vi "ScaleWayPoints_USB7855R.vi"(8 "AO Calibration Constants":cluster{"LSB Weight":u32, "Offset":i32}[](array[cluster]), 11 "WayPointCluster":T2) -> (0 "FPGA Way Points":i16[](array[numeric]), 2 "VelScallerCluster":T1, 3 ".not. x?":bool)   [LabVIEW 2023]
uses:
  TypeDefs/WayPointCluster.ctl
  TypeDefs/VelScallerCluster.ctl
  User_Vi/Settings.vi
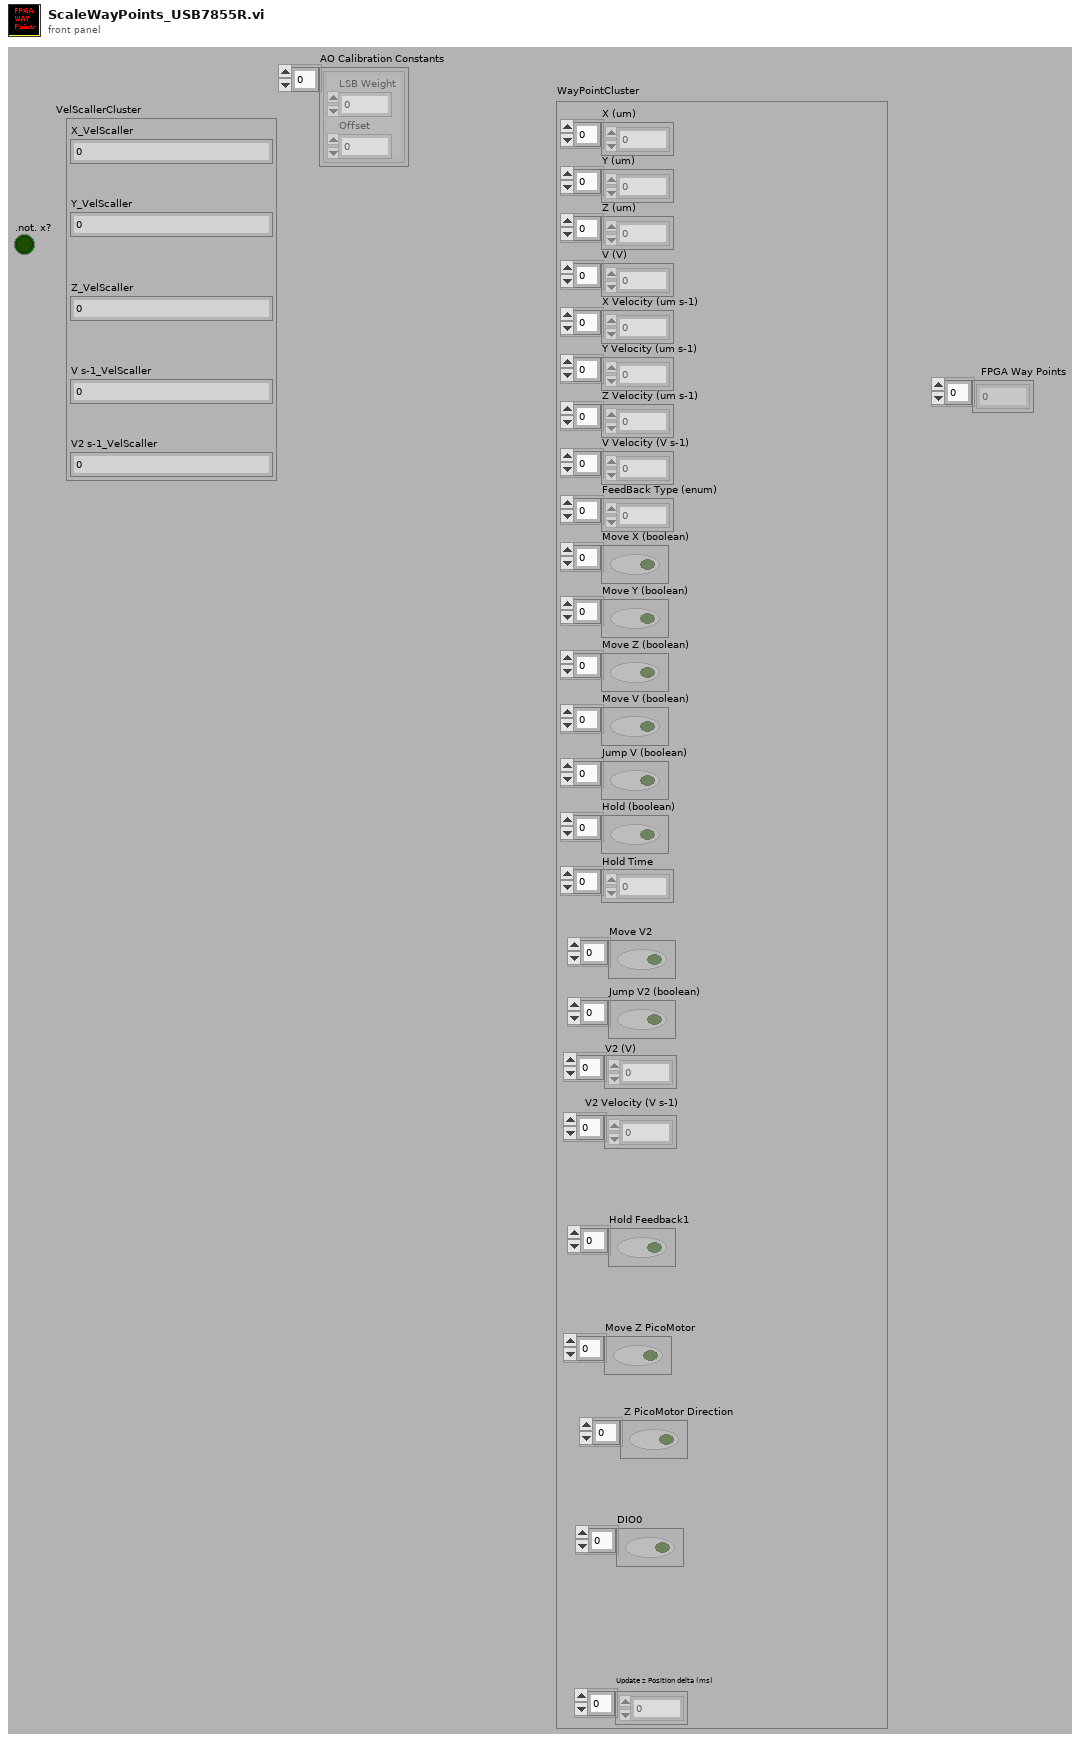
[diagram p1: front panel]
types:
  T1 = typedef "VelScallerCluster.ctl" = cluster{"X_VelScaller":i32, "Y_VelScaller":i32, "Z_VelScaller":i32, "V s-1_VelScaller":i32, "V2 s-1_VelScaller":i32}
  T2 = typedef "WayPointCluster.ctl" = cluster{"X (um)":dbl[], "Y (um)":dbl[], "Z (um)":dbl[], "V (V)":dbl[], "X Velocity (um s-1)":dbl[], "Y Velocity (um s-1)":dbl[], "Z Velocity (um s-1)":dbl[], "V Velocity (V s-1)":dbl[], "FeedBack Type (enum)":u16[], "Move X (boolean)":bool[], "Move Y (boolean)":bool[], "Move Z (boolean)":bool[], "Move V (boolean)":bool[], "Jump V (boolean)":bool[], "Hold (boolean)":bool[], "Hold Time":u32[], "V2 (V)":dbl[], "Move V2":bool[], "V2 Velocity (V s-1)":dbl[], "Jump V2 (boolean)":bool[], "Update z Position delta (ms)":i16[], "Hold Feedback1":bool[], "Move Z PicoMotor":bool[], " Z PicoMotor Direction":bool[], "DIO0":bool[]}
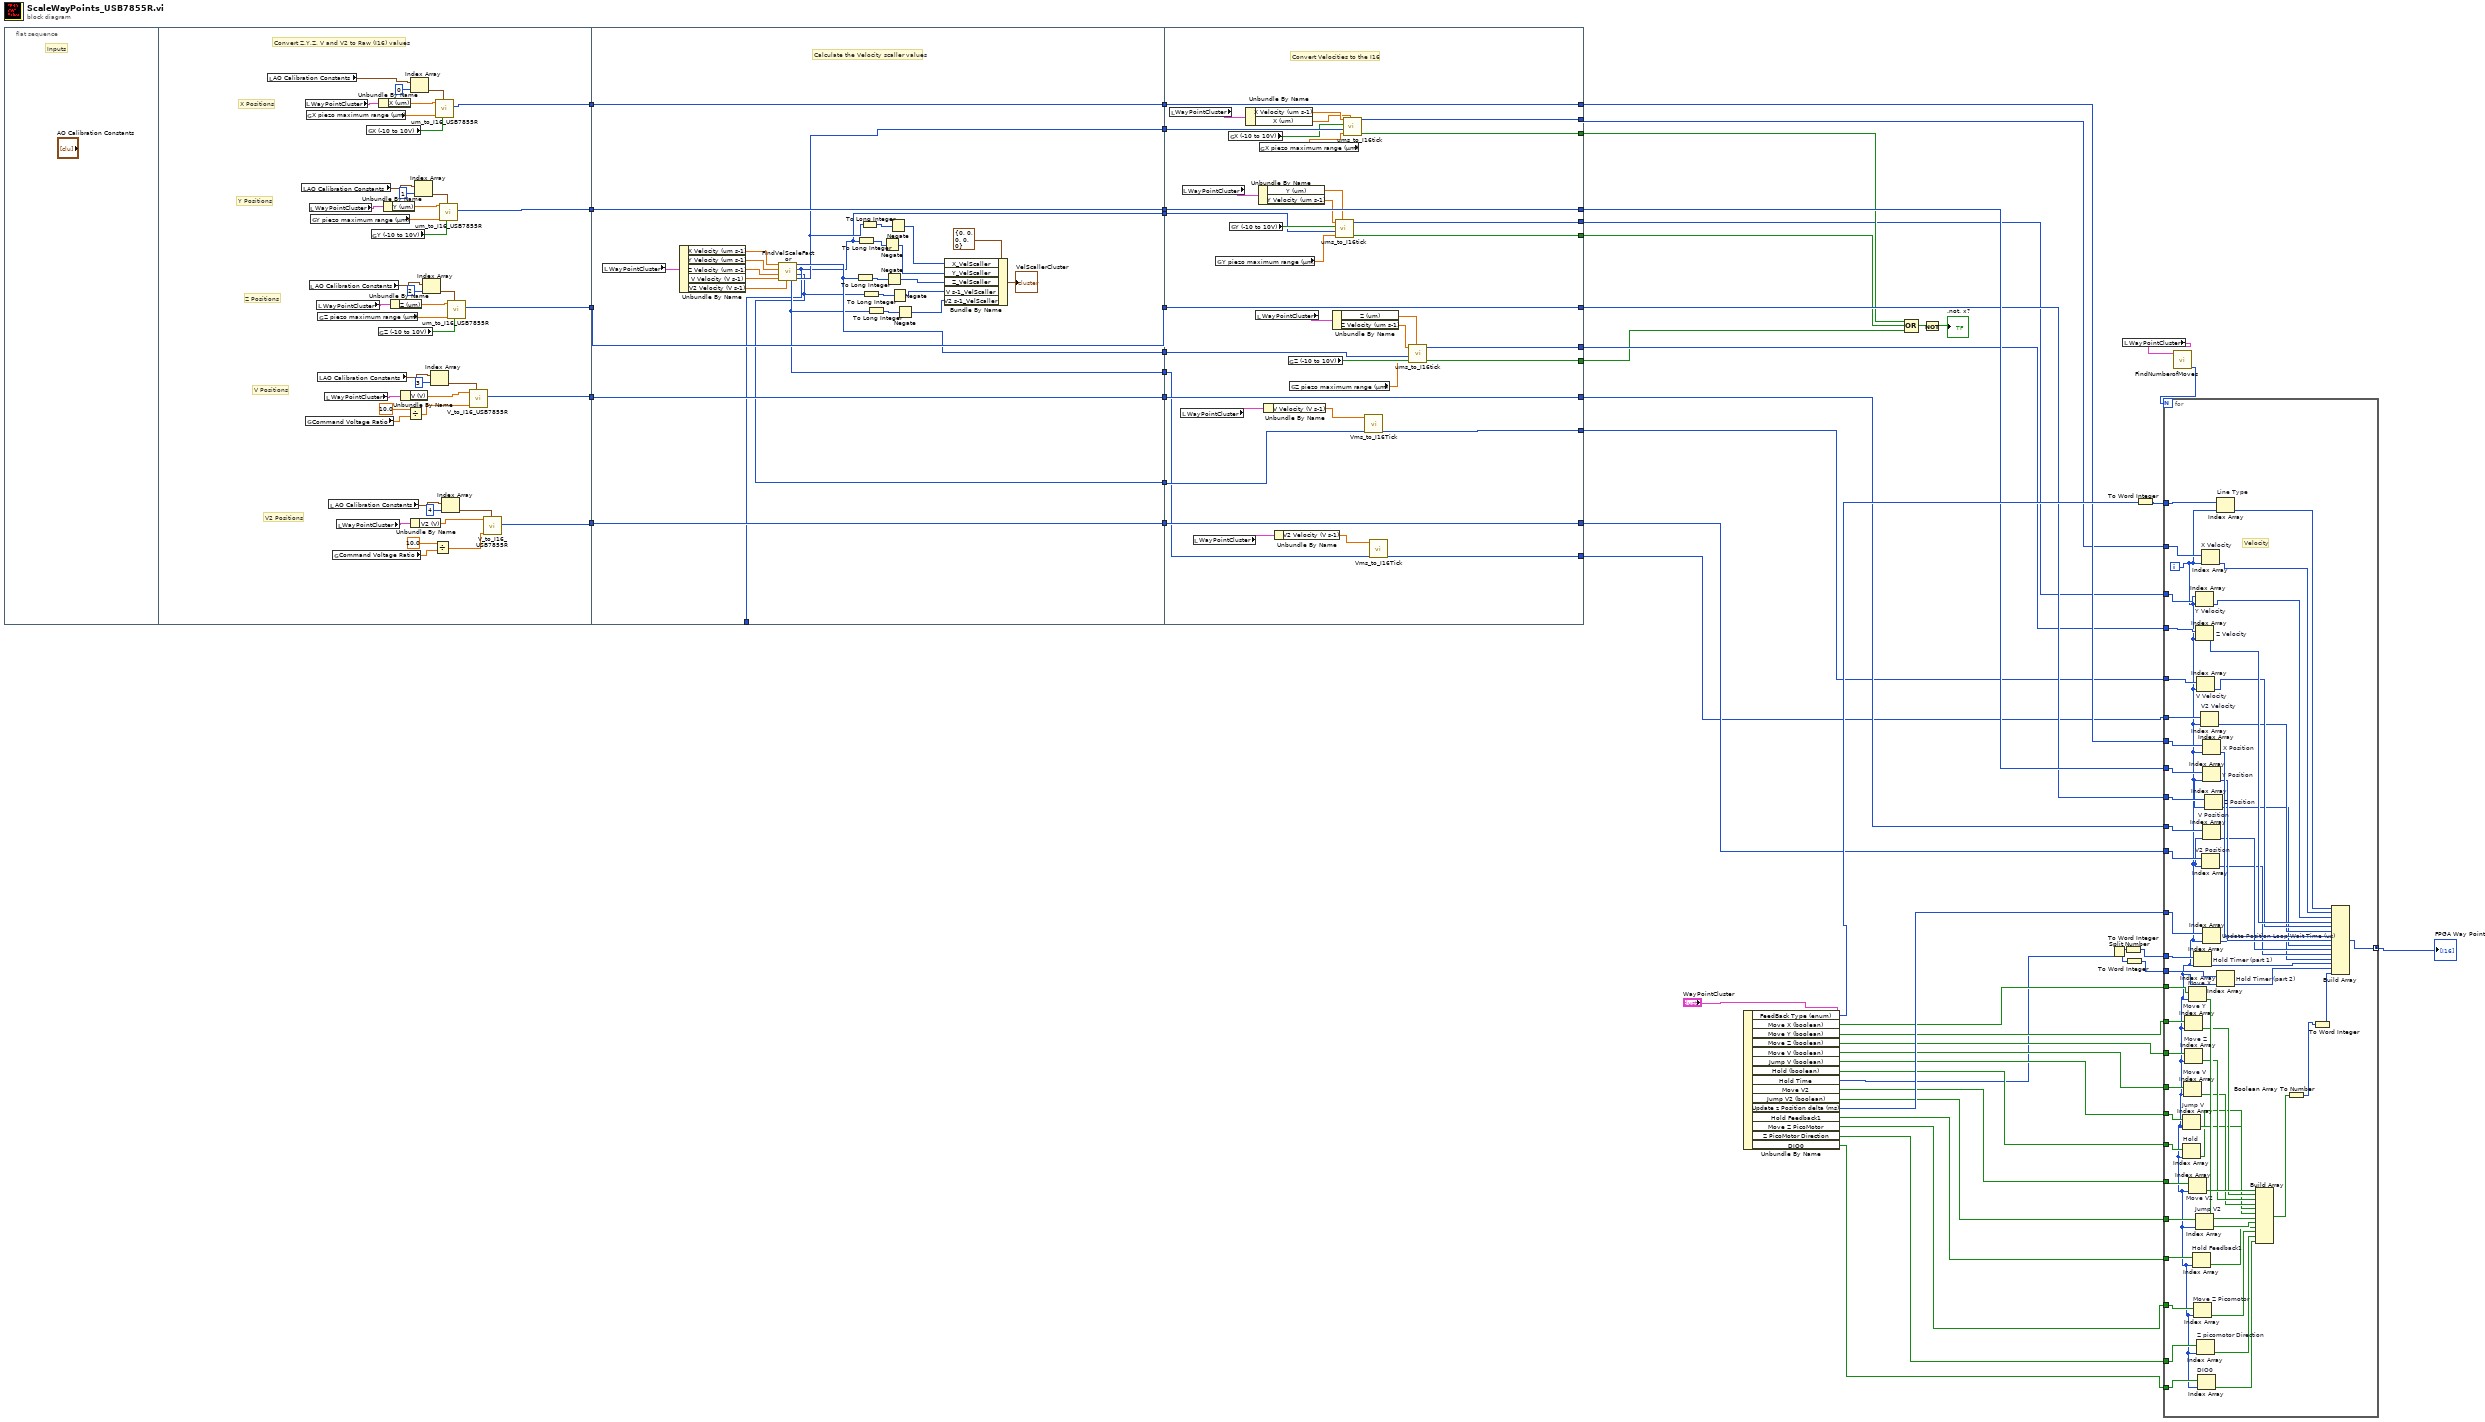
[diagram p0: block diagram]
diagram:
  n1 = flat-sequence {
    tunnel: [w96] -> w25
    tunnel: [w81] -> w24
    tunnel: [w73] -> w23
    tunnel: [w61] -> w22
    tunnel: [w55] -> w21
    tunnel: w25 -> [w124]
    tunnel: w24 -> [w123]
    tunnel: w23 -> [w122]
    tunnel: w22 -> [w121]
    tunnel: w21 -> [w120]
    tunnel: [w98] -> _
    tunnel: [w124] -> w20
    tunnel: [w123] -> w19
    tunnel: [w122] -> w18
    tunnel: [w121] -> w17
    tunnel: [w120] -> w16
    tunnel: [w119] -> w15
    tunnel: [w118] -> w14
    tunnel: [w99] -> w11
    tunnel: [w98] -> w10
    tunnel: [w97] -> w4
    tunnel: [w157] -> w26
    tunnel: [w158] -> w27
    tunnel: [w159] -> w28
    tunnel: [w160] -> w29
    tunnel: [w161] -> w30
    tunnel: w20 -> [w161]
    tunnel: w19 -> [w160]
    tunnel: w18 -> [w159]
    tunnel: w17 -> [w158]
    tunnel: w16 -> [w157]
    tunnel: w15 -> [w135]
    tunnel: w14 -> [w128]
    tunnel: [w156] -> w13
    tunnel: [w155] -> w12
    tunnel: w11 -> [w154]
    tunnel: w10 -> [w143]
    tunnel: [w142] -> w8
    tunnel: [w141] -> w9
    tunnel: [w134] -> w6
    tunnel: [w133] -> w7
    tunnel: [w132] -> w5
    tunnel: w4 -> [w129]
    tunnel: [w127] -> w3
    frame #0 {
      # "Inputs"
    }
    frame #1 {
      # "V2 Positions"
      # "V Positions"
      # "Z Positions"
      # "Y Positions"
      # "X Positions"
      # "Convert Z,Y,Z, V and V2 to Raw (I16) values"
      n2 = local read "AO Calibration Constants"() -> (w92:cluster{"LSB Weight":u32, "Offset":i32}[])
      n3 = local read "AO Calibration Constants"() -> (w85:cluster{"LSB Weight":u32, "Offset":i32}[])
      n4 = local read "WayPointCluster"() -> (w94:T2)
      n5 = global read "Settings.vi" "Command Voltage Ratio"() -> (w63:dbl)
      n6 = global read "Settings.vi" "X piezo maximum range (µm)"() -> (w95:dbl)
      n7 = local read "WayPointCluster"() -> (w83:T2)
      n8 = local read "AO Calibration Constants"() -> (w77:cluster{"LSB Weight":u32, "Offset":i32}[])
      n9 = global read "Settings.vi" "Y piezo maximum range (µm)"() -> (w82:dbl)
      n10 = local read "WayPointCluster"() -> (w79:T2)
      n11 = local read "AO Calibration Constants"() -> (w71:cluster{"LSB Weight":u32, "Offset":i32}[])
      n12 = global read "Settings.vi" "Z piezo maximum range (µm)"() -> (w80:dbl)
      n13 = local read "WayPointCluster"() -> (w70:T2)
      n14 = local read "AO Calibration Constants"() -> (w68:cluster{"LSB Weight":u32, "Offset":i32}[])
      n15 = global read "Settings.vi" "Command Voltage Ratio"() -> (w58:dbl)
      n16 = local read "WayPointCluster"() -> (w69:T2)
      n17 = global read "Settings.vi" "X (-10 to 10V)"() -> (w89:bool)
      n18 = global read "Settings.vi" "Y (-10 to 10V)"() -> (w88:bool)
      n19 = global read "Settings.vi" "Z (-10 to 10V)"() -> (w74:bool)
      n20 = Unbundle By Name(w94) -> ("X (um)"=w93:dbl[])
      n21 = Unbundle By Name(w83) -> ("Y (um)"=w84:dbl[])
      n22 = Unbundle By Name(w79) -> ("Z (um)"=w78:dbl[])
      n23 = Unbundle By Name(w70) -> ("V (V)"=w65:dbl[])
      n24 = Divide(x=10.0 ("Max/Min Value [V]"), y=w63) -> (x/y=w62:dbl)
      n25 = Index Array(array=w92, index=0) -> (element=w90:cluster{"LSB Weight":u32, "Offset":i32})
      n26 = Unbundle By Name(w69) -> ("V2 (V)"=w59:dbl[])
      n27 = Index Array(array=w85, index=1) -> (element=w87:cluster{"LSB Weight":u32, "Offset":i32})
      n28 = Index Array(array=w77, index=2) -> (element=w75:cluster{"LSB Weight":u32, "Offset":i32})
      n29 = Index Array(array=w71, index=3) -> (element=w66:cluster{"LSB Weight":u32, "Offset":i32})
      n30 = Divide(x=10.0 ("Max/Min Value [V]"), y=w58) -> (x/y=w56:dbl)
      n31 = call "um_to_I16_USB7855R.vi"("-10 to 10V?"=w89, "Calibration Constant"=w90, "Max Value [um]"=w95, "Input"=w93) -> ("Array"=w96:i16[])  [unwired: 7 in]
      n32 = call "um_to_I16_USB7855R.vi"("-10 to 10V?"=w88, "Calibration Constant"=w87, "Max Value [um]"=w82, "Input"=w84) -> ("Array"=w81:i16[])  [unwired: 7 in]
      n33 = Index Array(array=w68, index=4) -> (element=w60:cluster{"LSB Weight":u32, "Offset":i32})
      n34 = call "um_to_I16_USB7855R.vi"("-10 to 10V?"=w74, "Calibration Constant"=w75, "Max Value [um]"=w80, "Input"=w78) -> ("Array"=w73:i16[])  [unwired: 7 in]
      n35 = call "V_to_I16_USB7855R.vi"("Calibration Constant"=w66, "Max/Min Value [V]"=w62, "Input"=w65) -> ("16bit integer"=w61:i16[])  [unwired: 8 in]
      n36 = call "V_to_I16_USB7855R.vi"("Calibration Constant"=w60, "Max/Min Value [V]"=w56, "Input"=w59) -> ("16bit integer"=w55:i16[])  [unwired: 8 in]
    }
    frame #2 {
      # "Calculate the Velocity scaller values"
      n37 = local read "WayPointCluster"() -> (w117:T2)
      n38 = Unbundle By Name(w117) -> ("X Velocity (um s-1)"=w116:dbl[], "Y Velocity (um s-1)"=w115:dbl[], "Z Velocity (um s-1)"=w114:dbl[], "V Velocity (V s-1)"=w113:dbl[], "V2 Velocity (V s-1)"=w112:dbl[])
      n39 = call "FindVelScaleFactor.vi"("V2 Velocity [V s-1]"=w112, "V Velocity [V s-1]"=w113, "Z Velocity [um s-1]"=w114, "Y Velocity [um s-1]"=w115, "X Velocity [um s-1]"=w116) -> ("X_VelScaller"=w99:u32, "V s-1_VelScaller"=w97:u32, "Y_VelScaller"=w98:u32, "Z_VelScaller"=w119:u32, "V2 s-1_VelScaller"=w118:u32)  [unwired: 2 in]
      n40 = To Long Integer(number=w119) -> (32bit integer=w104:i32)
      n41 = To Long Integer(number=w98) -> (32bit integer=w103:i32)
      n42 = To Long Integer(number=w99) -> (32bit integer=w101:i32)
      n43 = To Long Integer(number=w97) -> (32bit integer=w102:i32)
      n44 = To Long Integer(number=w118) -> (32bit integer=w105:i32)
      n45 = Negate(x=w103) -> (-x=w108:i32)
      n46 = Negate(x=w104) -> (-x=w109:i32)
      n47 = Negate(x=w101) -> (-x=w106:i32)
      n48 = Negate(x=w102) -> (-x=w107:i32)
      n49 = Negate(x=w105) -> (-x=w110:i32)
      n50 = Bundle By Name(cluster=T1 {"X_VelScaller"=0, "Y_VelScaller"=0, "Z_VelScaller"=0, "V s-1_VelScaller"=0, "V2 s-1_VelScaller"=0} ("VelScallerCluster"), "X_VelScaller"=w106, "Y_VelScaller"=w108, "Z_VelScaller"=w109, "V s-1_VelScaller"=w107, "V2 s-1_VelScaller"=w110) -> (→"VelScallerCluster":T1)
    }
    frame #3 {
      # "Convert Velocities to the I16"
      n51 = local read "WayPointCluster"() -> (w151:T2)
      n52 = local read "WayPointCluster"() -> (w131:T2)
      n53 = local read "WayPointCluster"() -> (w146:T2)
      n54 = local read "WayPointCluster"() -> (w126:T2)
      n55 = global read "Settings.vi" "Y piezo maximum range (µm)"() -> (w148:dbl)
      n56 = global read "Settings.vi" "X (-10 to 10V)"() -> (w152:bool)
      n57 = global read "Settings.vi" "Y (-10 to 10V)"() -> (w147:bool)
      n58 = Unbundle By Name(w151) -> ("X Velocity (um s-1)"=w150:dbl[], "X (um)"=w149:dbl[])
      n59 = local read "WayPointCluster"() -> (w138:T2)
      n60 = Unbundle By Name(w146) -> ("Y (um)"=w145:dbl[], "Y Velocity (um s-1)"=w144:dbl[])
      n61 = global read "Settings.vi" "X piezo maximum range (µm)"() -> (w153:dbl)
      n62 = Unbundle By Name(w131) -> ("V Velocity (V s-1)"=w130:dbl[])
      n63 = Unbundle By Name(w126) -> ("V2 Velocity (V s-1)"=w125:dbl[])
      n64 = global read "Settings.vi" "Z (-10 to 10V)"() -> (w137:bool)
      n65 = global read "Settings.vi" "Z piezo maximum range (µm)"() -> (w136:dbl)
      n66 = Unbundle By Name(w138) -> ("Z (um)"=w139:dbl[], "Z Velocity (um s-1)"=w140:dbl[])
      n67 = call "ums_to_I16tick.vi"("Positions"=w145, "Max piezo distance"=w148, "n"=w143, "-10 to +10V?"=w147, "Input Velocity"=w144) -> ("Error"=w142:bool, "Scalled Velocity"=w141:i16[])  [unwired: 3 in]
      n68 = call "ums_to_I16tick.vi"("Positions"=w149, "Max piezo distance"=w153, "n"=w154, "-10 to +10V?"=w152, "Input Velocity"=w150) -> ("Error"=w156:bool, "Scalled Velocity"=w155:i16[])  [unwired: 3 in]
      n69 = call "Vms_to_I16Tick.vi"("n"=w129, "V Velocity [V s-1]"=w130) -> ("V Velocity"=w132:i16[])  [unwired: 9 in]
      n70 = call "Vms_to_I16Tick.vi"("n"=w128, "V Velocity [V s-1]"=w125) -> ("V Velocity"=w127:i16[])  [unwired: 9 in]
      n71 = call "ums_to_I16tick.vi"("Positions"=w139, "Max piezo distance"=w136, "n"=w135, "-10 to +10V?"=w137, "Input Velocity"=w140) -> ("Error"=w134:bool, "Scalled Velocity"=w133:i16[])  [unwired: 3 in]
    }
  }
  n72 = Unbundle By Name("WayPointCluster") -> ("FeedBack Type (enum)"=w39:u16[], "Move X (boolean)"=w49:bool[], "Move Y (boolean)"=w48:bool[], "Move Z (boolean)"=w47:bool[], "Move V (boolean)"=w46:bool[], "Jump V (boolean)"=w45:bool[], "Hold (boolean)"=w44:bool[], "Hold Time"=w37:u32[], "Move V2"=w43:bool[], "Jump V2 (boolean)"=w42:bool[], "Update z Position delta (ms)"=w50:i16[], "Hold Feedback1"=w40:bool[], "Move Z PicoMotor"=w36:bool[], "Z PicoMotor Direction"=w35:bool[], "DIO0"=w1:bool[])
  n73 = Compound Arithmetic op=OR(w13, w8, w6) -> (w53:bool)
  n74 = Not(x=w53) -> (.not. x?=→".not. x?":bool)
  n75 = Split Number(x=w37) -> (hi(x)=w34:u16[], lo(x)=w32:u16[])
  n76 = local read "WayPointCluster"() -> (w2:T2)
  n77 = To Word Integer(number=w34) -> (16bit integer=w33:i16[])
  n78 = To Word Integer(number=w32) -> (16bit integer=w31:i16[])
  n79 = To Word Integer(number=w39) -> (16bit integer=w38:i16[])
  n80 = call "FindNumberofMoves.vi"("WayPointCluster"=w2) -> ("max length"=w51:i32)  [unwired: 10 in]
  n81 = for {
    N: w51 -> [_]
    tunnel: w5 -> [w215]
    tunnel: w7 -> [w216]
    tunnel: w9 -> [w217]
    tunnel: w12 -> [w218]
    tunnel: [w213] -> w41 mode=concatenating
    tunnel: w3 -> [w209]
    tunnel: w30 -> [w207]
    tunnel: w29 -> [w205]
    tunnel: w28 -> [w203]
    tunnel: w27 -> [w201]
    tunnel: w26 -> [w199]
    tunnel: w38 -> [w197]
    tunnel: w50 -> [w196]
    tunnel: w33 -> [w194]
    tunnel: w49 -> [w191]
    tunnel: w48 -> [w189]
    tunnel: w47 -> [w187]
    tunnel: w46 -> [w185]
    tunnel: w45 -> [w183]
    tunnel: w44 -> [w181]
    tunnel: w43 -> [w179]
    tunnel: w42 -> [w177]
    tunnel: w40 -> [w175]
    tunnel: w36 -> [w170]
    tunnel: w35 -> [w169]
    tunnel: w31 -> [w165]
    tunnel: w1 -> [w164]
    i -> [w163]
    # "Velocity"
    n82 = Index Array "Jump V"(array=w183, index=w163) -> (element=w182:bool)
    n83 = Index Array "Hold"(array=w181, index=w163) -> (element=w180:bool)
    n84 = Index Array "Move V"(array=w185, index=w163) -> (element=w184:bool)
    n85 = Index Array "Move Y"(array=w189, index=w163) -> (element=w188:bool)
    n86 = Index Array "Move Z"(array=w187, index=w163) -> (element=w186:bool)
    n87 = Index Array "Move V2"(array=w179, index=w163) -> (element=w178:bool)
    n88 = Index Array "Move X"(array=w191, index=w163) -> (element=w190:bool)
    n89 = Index Array "Hold Feedback1"(array=w175, index=w163) -> (element=w174:bool)
    n90 = Index Array "Hold Timer (part 1)"(array=w194, index=w163) -> (element=w193:i16)
    n91 = Index Array "Move Z Picomotor"(array=w170, index=w163) -> (element=w168:bool)
    n92 = Index Array "Y Velocity"(array=w217, index=w163) -> (element=w212:i16)
    n93 = Index Array "Jump V2"(array=w177, index=w163) -> (element=w176:bool)
    n94 = Index Array "Z Velocity"(array=w216, index=w163) -> (element=w211:i16)
    n95 = Index Array "V Velocity"(array=w215, index=w163) -> (element=w210:i16)
    n96 = Index Array "Z picomotor Direction"(array=w169, index=w163) -> (element=w167:bool)
    n97 = Index Array "DIO0"(array=w164, index=w163) -> (element=w162:bool)
    n98 = Index Array "V2 Velocity"(array=w209, index=w163) -> (element=w208:i16)
    n99 = Index Array "X Velocity"(array=w218, index=w163) -> (element=w214:i16)
    n100 = Index Array "V2 Position"(array=w199, index=w163) -> (element=w198:i16)
    n101 = Index Array "Y Position"(array=w205, index=w163) -> (element=w204:i16)
    n102 = Index Array "Update Position Loop Wait Time (us)"(array=w196, index=w163) -> (element=w195:i16)
    n103 = Index Array "X Position"(array=w207, index=w163) -> (element=w206:i16)
    n104 = Index Array "V Position"(array=w201, index=w163) -> (element=w200:i16)
    n105 = Index Array "Z Position"(array=w203, index=w163) -> (element=w202:i16)
    n106 = Index Array "Hold Timer (part 2)"(array=w165, index=w163) -> (element=w166:i16)
    n107 = Index Array "Line Type"(array=w197, index=w163) -> (element=w171:i16)
    n108 = Build Array(w190, w188, w186, w184, w182, w180, w178, w176, w174, w168, w167, w162) -> (w192:bool[])
    n109 = Boolean Array To Number(Boolean array=w192) -> (number=w173:u16)
    n110 = To Word Integer(number=w173) -> (16bit integer=w172:i16)
    n111 = Build Array(w171, w214, w212, w211, w210, w208, w206, w204, w202, w200, w198, w195, w193, w166, w172) -> (w213:i16[])
  }
  "FPGA Way Points" <- w41
